vi "support_getAppDir.vi"(8 "error in (no error)":errorcluster) -> (0 "error out":errorcluster, 3 "App.Dir":path)   [LabVIEW 2015]
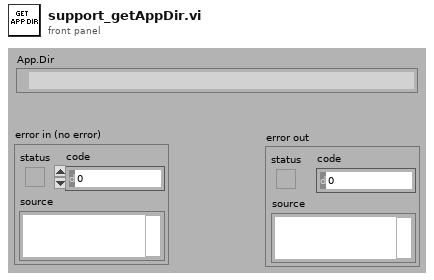
[diagram p1: front panel]
types:
  T1 = enum32{"invalid app kind", "Development System", "Run Time System", "Student Edition", "Embedded LabVIEW", "Evaluation", "Custom"}
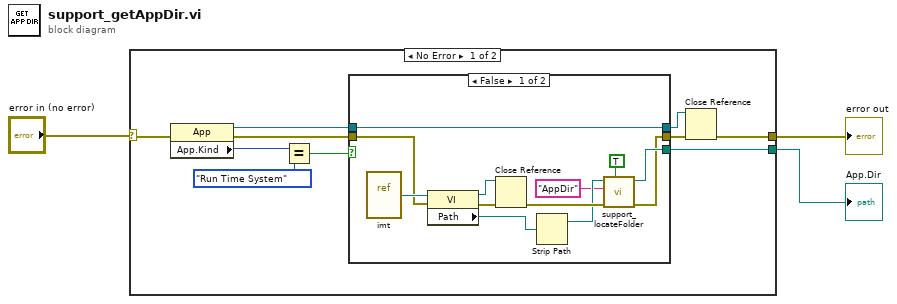
[diagram p0: block diagram]
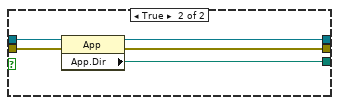
[diagram p2: hidden frame]
diagram:
  n1 = case shown="No Error" "error in (no error)" {
    selector: "error in (no error)" -> [w13 w31]
    tunnel: [w5 w31] -> w1
    tunnel: [w4 _] -> w2
    frame No Error {
      n2 = property class="App"(error in=w13) -> (reference out=w8:refnum<vi>, error out=w9:errorcluster, "App.Kind"=w12:T1)  [unwired: 1 in]
      n3 = Equal?(x=w12, y=T1."Run Time System") -> (x = y?=w10:bool)
      n4 = case shown="False" w10 {
        tunnel: w9 -> [w23 w29]
        tunnel: w8 -> [w25 w30]
        tunnel: [w25 w28] -> w6
        tunnel: [w14 w27] -> w7
        tunnel: [w15 w26] -> w4
        frame False {
          n5 = vi-ref "imt.vi"() -> (w24:refnum<vi>)
          n6 = property class="VI"(reference=w24, error in=w23) -> (reference out=w21:refnum<vi>, error out=w22:errorcluster, "Path"=w20:path)
          n7 = Close Reference(reference=w21, error in (no error)=w22) -> (error out=w19:errorcluster)
          n8 = Strip Path(path=w20) -> (stripped path=w18:path)  [unwired: 1 out]
          n9 = call "support_locateFolder.vi"("create if not found?"=TRUE, "error in (no error)"=w19, "Folder"="AppDir", "Root"=w18) -> ("error IO"=w14:errorcluster, "path"=w15:path)  [unwired: 5 in, 1 out]
        }
        frame True {
          n10 = property class="App"(reference=w30, error in=w29) -> (reference out=w28:refnum<vi>, error out=w27:errorcluster, "App.Dir"=w26:path)
        }
      }
      n11 = Close Reference(reference=w6, error in (no error)=w7) -> (error out=w5:errorcluster)
    }
    frame Error {
    }
  }
  "App.Dir" <- w2
  "error out" <- w1
